vi "LQG_Host.vi"() -> ()   [LabVIEW 2022 SP3]
uses:
  <vilib>/rvi/interface/nirviMethod/nirviMethod.xnode
  <vilib>/rvi/errors/niLvFpgaMergeErrorWithErrorCode.vi
  <vilib>/FPGAPlugInAG/Dynamic/niLvFpga_Reset_Dynamic.vi
  <vilib>/FPGAPlugInAG/Dynamic/niLvFpga_Run_Dynamic.vi
  <vilib>/rvi/interface/nirviOpenFPGA/nirviOpenFPGA.xnode
  <vilib>/FPGAPlugInAG/Dynamic/niLvFpga_WriteFifo_Dynamic.vi
  <vilib>/FPGAPlugInAG/Dynamic/niLvFpga_ReadFifo_Dynamic.vi
  FPGA Bitfiles/lqgcontrollerpro_FPGATarget_LQGTarget_BqkXz-HMbBs.lvbitx
  LQG_Target.vi
  <vilib>/FPGAPlugInAG/cRIO-9054/niLvFpga_Open_cRIO-9054.vi
  <vilib>/rvi/interface/common/dynamic/niFpgaDynamicAddResources.vi
panel:
  out "Numeric":i32
  out "Controlled Force":sgl[](graph)
  out "Uncontrolled Displacement":dynamicdata(graph)
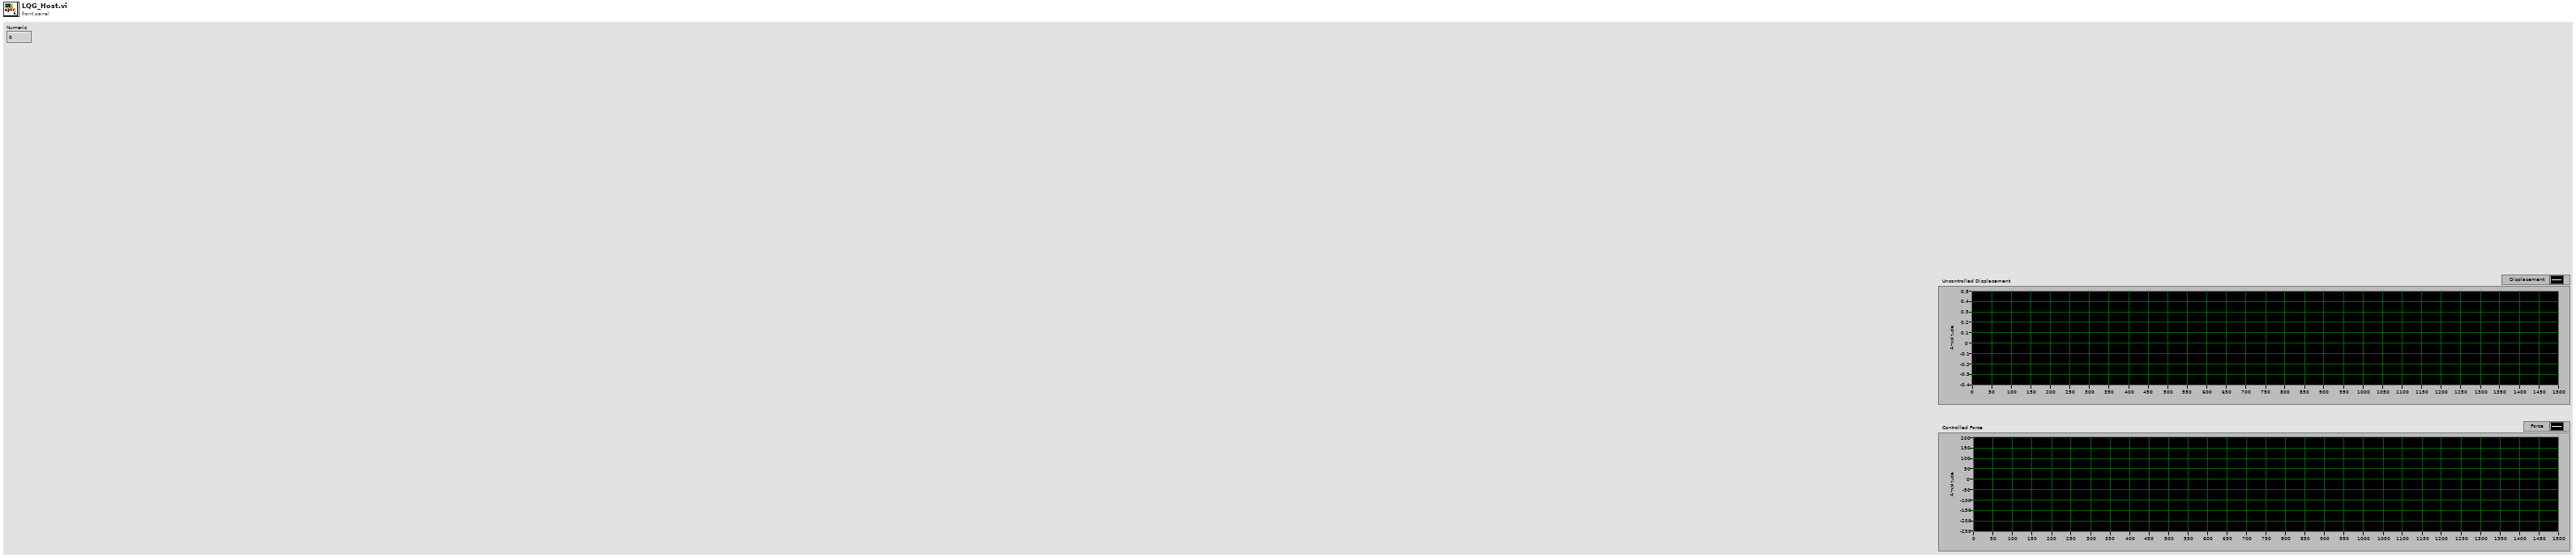
[diagram p1: front panel]
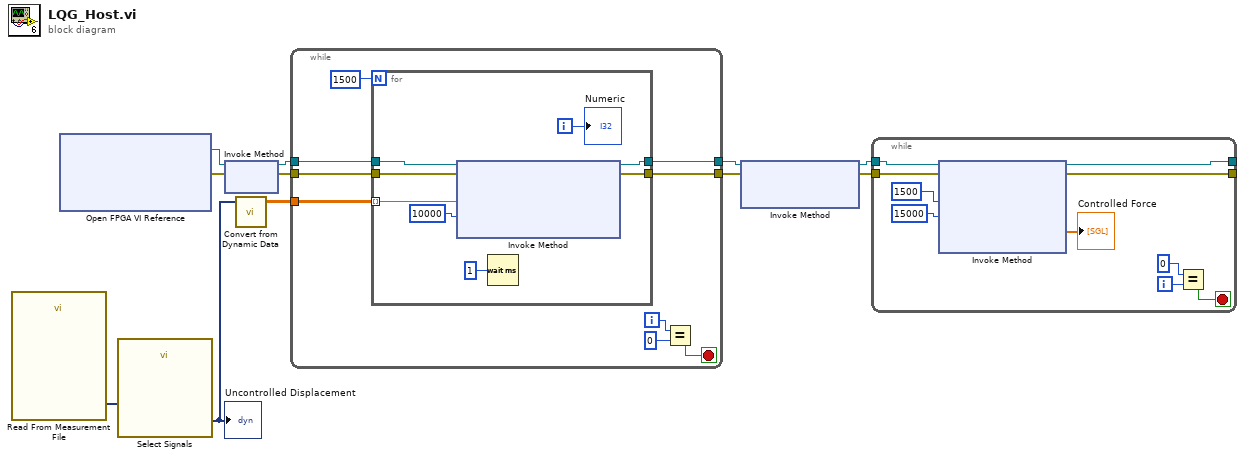
[diagram p0: block diagram]
diagram:
  n1 = call "Read From Measurement File"() -> ("Signals"=w3:dynamicdata)  [unwired: 6 in, 5 out]
  n2 = xnode "Open FPGA VI Reference"() -> ("FPGA VI Reference Out"=w2:refnum<k20>, "error out"=w1:errorcluster)  [unwired: 2 in]
  n3 = call "Select Signals"("Signals"=w3) -> ("Signal Out"=w11:dynamicdata)  [unwired: 9 in, 1 out]
  "Uncontrolled Displacement" <- w11
  n4 = xnode "Invoke Method"("FPGA VI Reference In"=w2, "error in"=w1) -> ("FPGA VI Reference Out"=w10:refnum<k20>, "error out"=w8:errorcluster)
  n5 = call "Convert from Dynamic Data"("Dynamic Data Type"=w11) -> ("Array"=w4:dbl[][])  [unwired: 3 in]
  n6 = while {
    tunnel: w4 -> [w19]
    tunnel: w10 -> [w18]
    tunnel: [w16] -> w6
    tunnel: w8 -> [w13]
    tunnel: [w12] -> w5
    i -> [w14]
    stop <- w17 stop-if-true
    n7 = for {
      N: 1500 -> [_]
      tunnel: w19 -> [w25] mode=indexing
      tunnel: w18 -> [w26]
      tunnel: [w24] -> w16
      tunnel: w13 -> [w22]
      tunnel: [w21] -> w12
      i -> [w23]
      n8 = xnode "Invoke Method"("FPGA VI Reference In"=w26, "error in"=w22, "Data"=w25, "Timeout (ms)"=10000) -> ("FPGA VI Reference Out"=w24:refnum<k20>, "error out"=w21:errorcluster)  [unwired: 1 out]
      n9 = Wait (ms)(milliseconds to wait=u32 1) -> ()  [unwired: 1 out]
      "Numeric" <- w23
    }
    n10 = Equal?(x=w14, y=u32 0) -> (x = y?=w17:bool)
  }
  n11 = xnode "Invoke Method"("FPGA VI Reference In"=w6, "error in"=w5) -> ("FPGA VI Reference Out"=w9:refnum<k20>, "error out"=w7:errorcluster)  [unwired: 1 in]
  n12 = while {
    tunnel: [w37] -> _
    tunnel: w9 -> [w35]
    tunnel: w7 -> [w30]
    tunnel: [w29] -> _
    i -> [w34]
    stop <- w32 stop-if-true
    n13 = xnode "Invoke Method"("FPGA VI Reference In"=w35, "error in"=w30, "Number of Elements"=u32 1500, "Timeout (ms)"=15000) -> ("FPGA VI Reference Out"=w37:refnum<k20>, "error out"=w29:errorcluster, "Data"=→"Controlled Force":sgl[])  [unwired: 1 out]
    n14 = Equal?(x=0, y=w34) -> (x = y?=w32:bool)
  }
